vi "I2C WriteRead Data.vi"(5 "Address":T2 format="%02x", 6 "NoStop (F)":bool, 7 "I2C #":T1=-1, 8 "error in (no error)":errorcluster, 9 "Len":u8, 10 "Write Data":string, 11 "Session in":refnum<class "Session.lvclass">) -> (0 "error out":errorcluster, 1 "Read Data":string, 3 "Session out":refnum<class "Session.lvclass">)   [LabVIEW 2025, in "CTI.lvlib" / "Session.lvclass"]
doc: "This VI can be useful for register style read operations that are common in many peripherals. Typically a register number is sent to the peripheral and then a set number of bytes are read back from the device corresponding to the register contents."
uses:
  Session.lvclass
  I2C Address.ctl
  I2C Number.ctl
  <vilib>/Utility/error.llb/Error Cluster From Error Code.vi
  <vilib>/ErrorRing/Error Ring.xnode
  Session.lvclass/Session.ctl
  DeviceComms/DeviceComms.lvclass
  CTI.lvlib
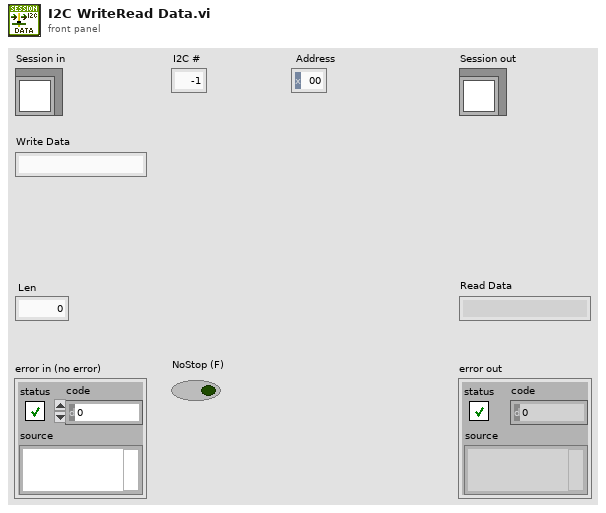
[diagram p1: front panel]
types:
  T1 = typedef "CTI.lvlib/I2C Number.ctl" = i8
  T2 = typedef "CTI.lvlib/I2C Address.ctl" = u8
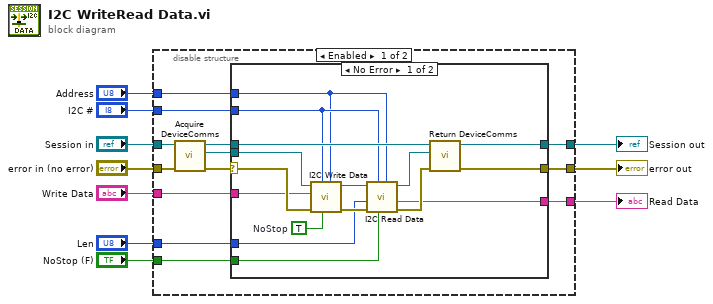
[diagram p0: block diagram]
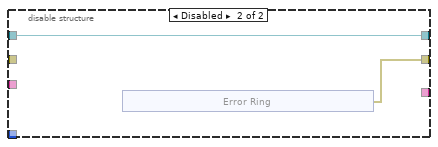
[diagram p3: hidden frame]
diagram:
  n1 = disable-structure shown="Enabled" {
    disable-tunnel: "Session in" -> [w20 w43]
    disable-tunnel: "error in (no error)" -> [w19 _]
    disable-tunnel: "I2C #" -> [w18 _]
    disable-tunnel: "Write Data" -> [w17 _]
    disable-tunnel: "Address" -> [w16 _]
    disable-tunnel: "Len" -> [w15 _]
    disable-tunnel: "NoStop (F)" -> [w14 _]
    disable-tunnel: [w13 w42] -> w3
    disable-tunnel: [w12 w43] -> w2
    disable-tunnel: [w11 _] -> w1
    frame Enabled {
      n2 = call "Acquire DeviceComms.vi"("error in (no error)"=w19, "Session in"=w20) -> ("error out"=w22:errorcluster, "DeviceComms"=w21:refnum<class "DeviceComms.lvclass">, "Session out"=w23:refnum<class "Session.lvclass">)  [unwired: 7 in]
      n3 = case shown="No Error" w22 {
        selector: w22 -> [w38 w41]
        tunnel: w23 -> [w37 w40]
        tunnel: w21 -> [w39 _]
        tunnel: [w35 w40] -> w12
        tunnel: [w34 w41] -> w13
        tunnel: w18 -> [w29 _]
        tunnel: w17 -> [w33 _]
        tunnel: w16 -> [w28 _]
        tunnel: w15 -> [w27 _]
        tunnel: w14 -> [w26 _]
        tunnel: [w24 _] -> w11
        frame No Error {
          w25 = TRUE  # NoStop
          n4 = call-dynamic "I2C Write Data.vi"("Address"=w28, "NoStop (F)"=w25, "I2C #"=w29, "error in (no error)"=w38, "Data"=w33, "DeviceComms in"=w39) -> ("error out"=w36:errorcluster, "DeviceComms out"=w31:refnum<class "DeviceComms.lvclass">)  [unwired: 4 in]
          n5 = call-dynamic "I2C Read Data.vi"("Address"=w28, "NoStop (F)"=w26, "I2C #"=w29, "error in (no error)"=w36, "Len"=w27, "DeviceComms in"=w31) -> ("error out"=w32:errorcluster, "Data"=w24:string, "DeviceComms out"=w30:refnum<class "DeviceComms.lvclass">)  [unwired: 3 in]
          n6 = call "Return DeviceComms.vi"("error in (no error)"=w32, "DeviceComms"=w30, "Session in"=w37) -> ("error out"=w34:errorcluster, "Session out"=w35:refnum<class "Session.lvclass">)  [unwired: 7 in]
        }
        frame Error {
        }
      }
    }
    frame Disabled {
      n7 = xnode "Error Ring"() -> ("error out"=w42:errorcluster)
    }
  }
  "error out" <- w3
  "Session out" <- w2
  "Read Data" <- w1
